vi "Write Sub Panel Msg.vi"(8 "error in (no error)":errorcluster, 10 "Sub Panel Msg":refnum<vi>, 11 "Messages Actor in":refnum<class "Messages Actor.lvclass">) -> (0 "error out":errorcluster, 3 "Messages Actor out":refnum<class "Messages Actor.lvclass">)   [LabVIEW 2020, in "Messages Actor.lvlib" / "Messages Actor.lvclass"]
uses:
  Messages Actor.lvclass
  Messages Actor.lvclass/Messages Actor.ctl
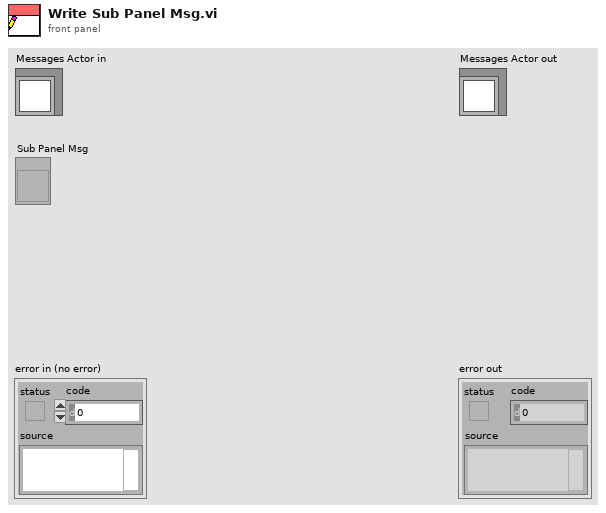
[diagram p1: front panel]
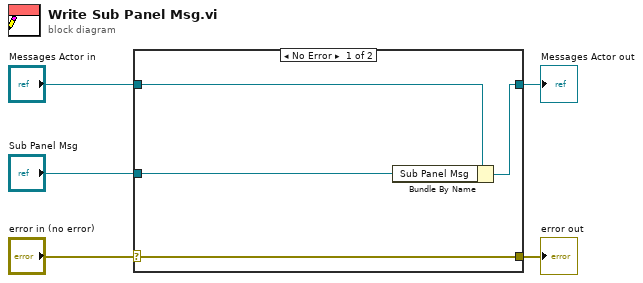
[diagram p0: block diagram]
diagram:
  n1 = case shown="No Error" "error in (no error)" {
    selector: "error in (no error)" -> [w9 w10]
    tunnel: [w9 w10] -> w4
    tunnel: [w7 w11] -> w2
    tunnel: "Messages Actor in" -> [w8 w11]
    tunnel: "Sub Panel Msg" -> [w6 _]
    frame No Error {
      n2 = Bundle By Name(cluster=w8, "Sub Panel Msg"=w6) -> (w7:refnum<class "Messages Actor.lvclass">)
    }
    frame Error {
    }
  }
  "error out" <- w4
  "Messages Actor out" <- w2
